vi "Configure Timer Trigger.vi"(0 "VISA resource name":refnum<visa-resource-name>, 1 "Seconds (0)":dbl, 2 "Generate Timer Event (F: Disable)":bool, 3 "Timer Delay (1E-5)":dbl=1e-05, 5 "Timer Number (1: Timer 1)":i32(ring)=1 items=["Timer 1"=1, "Timer 2"=2, "Timer 3"=3, "Timer 4"=4], 7 "Count (0)":u32, 9 "Timer Stimulus Event (\"NONE\")":string="NONE", 11 "error in (no error)":errorcluster, 12 "Fractional Seconds (0)":dbl, 13 "Enable Timer Trigger (F: Disable)":bool) -> (4 "VISA resource name out":refnum<visa-resource-name>, 15 "error out":errorcluster)   [LabVIEW 2016, in "Keithley DMM6500 DAQ6500 Series.lvlib"]
doc: "Configures the timer trigger."
uses:
  Keithley DMM6500 DAQ6500 Series.lvlib
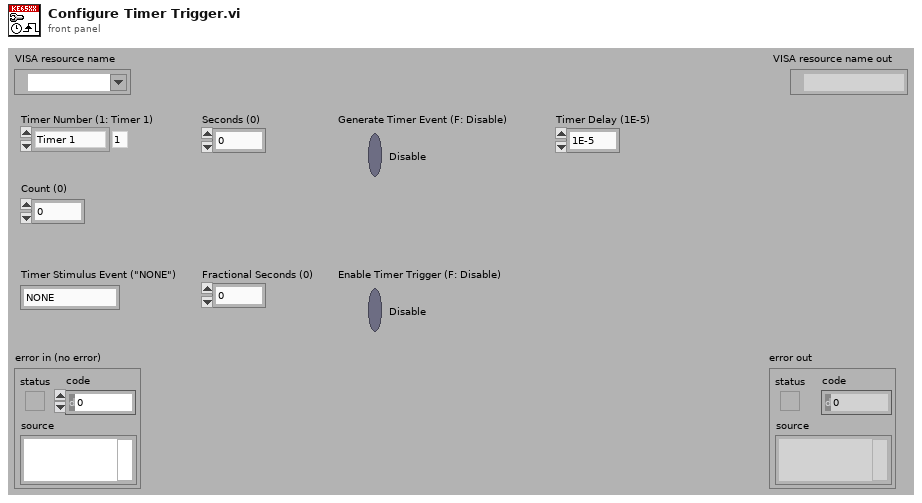
[diagram p1: front panel]
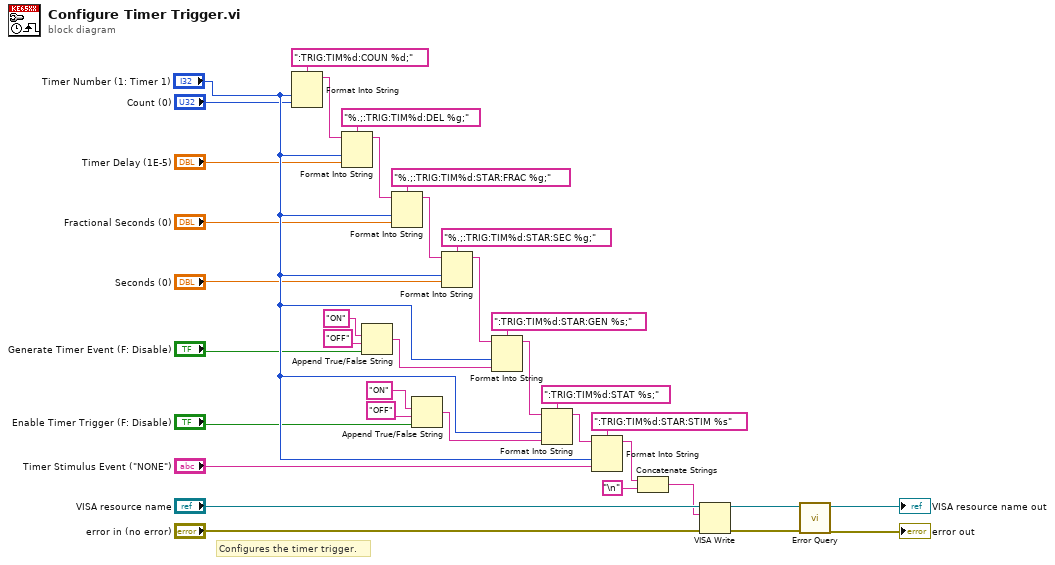
[diagram p0: block diagram]
diagram:
  # "Configures the timer trigger."
  n1 = Format Into String(format string=":TRIG:TIM%d:COUN %d;", "Timer Number (1: Timer 1)", "Count (0)") -> (resulting string=w33:string)  [unwired: 2 in, 1 out]
  n2 = Format Into String(format string="%.;:TRIG:TIM%d:DEL %g;", initial string=w33, "Timer Number (1: Timer 1)", "Timer Delay (1E-5)") -> (resulting string=w30:string)  [unwired: 1 in, 1 out]
  n3 = Append True/False String(1:"Generate Timer Event (F: Disable)", 2:"OFF", 3:"ON") -> (0:w19:string)  [unwired: 1 in]
  n4 = Format Into String(format string="%.;:TRIG:TIM%d:STAR:FRAC %g;", initial string=w30, "Timer Number (1: Timer 1)", "Fractional Seconds (0)") -> (resulting string=w27:string)  [unwired: 1 in, 1 out]
  n5 = Append True/False String(1:"Enable Timer Trigger (F: Disable)", 2:"OFF", 3:"ON") -> (0:w13:string)  [unwired: 1 in]
  n6 = Format Into String(format string="%.;:TRIG:TIM%d:STAR:SEC %g;", initial string=w27, "Timer Number (1: Timer 1)", "Seconds (0)") -> (resulting string=w21:string)  [unwired: 1 in, 1 out]
  n7 = Format Into String(format string=":TRIG:TIM%d:STAR:GEN %s;", initial string=w21, "Timer Number (1: Timer 1)", w19) -> (resulting string=w15:string)  [unwired: 1 in, 1 out]
  n8 = Format Into String(format string=":TRIG:TIM%d:STAT %s;", initial string=w15, "Timer Number (1: Timer 1)", w13) -> (resulting string=w12:string)  [unwired: 1 in, 1 out]
  n9 = Format Into String(format string=":TRIG:TIM%d:STAR:STIM %s", initial string=w12, "Timer Number (1: Timer 1)", "Timer Stimulus Event (\"NONE\")") -> (resulting string=w2:string)  [unwired: 1 in, 1 out]
  n10 = Concatenate Strings(w2, "\n") -> (w3:string)
  n11 = VISA Write(VISA resource name="VISA resource name", write buffer=w3, error in (no error)="error in (no error)") -> (VISA resource name out=w7:refnum<visa-resource-name>, error out=w6:errorcluster)  [unwired: 1 out]
  n12 = call "Error Query.vi"("error in (no error)"=w6, "VISA resource name"=w7) -> ("error out"=→"error out":errorcluster, "VISA resource name out"=→"VISA resource name out":refnum<visa-resource-name>)  [unwired: 6 in, 2 out]
